vi "FTW-Endpoint-TCP-Receive-Worker.vi"(0 "TCP Endpoint":refnum<class "FTW-Endpoint-TCP.lvclass">, 5 "Address":string) -> ()   [LabVIEW 2013, in "FTW-Endpoint-TCP.lvclass"]
uses:
  FTW-Endpoint-TCP.lvclass
  FTW-Endpoint-TCP.lvclass/FTW-Endpoint-TCP.ctl
panel:
  out "connected":bool
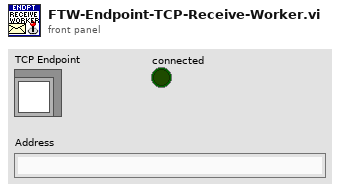
[diagram p1: front panel]
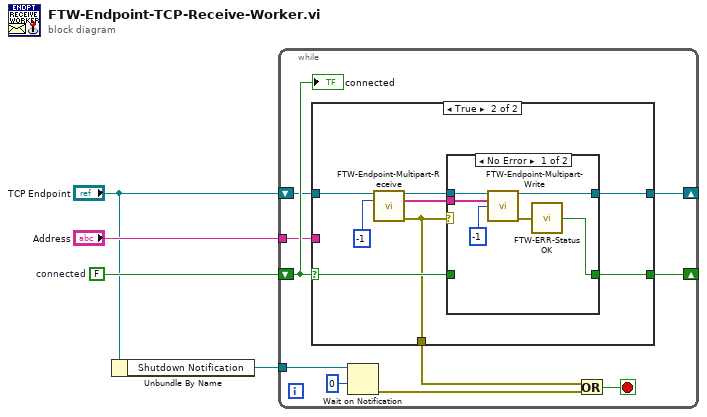
[diagram p0: block diagram]
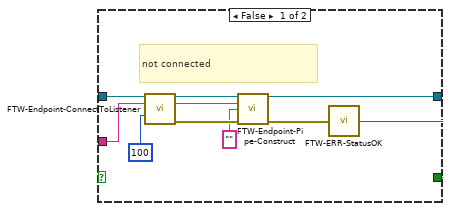
[diagram p2: hidden frame]
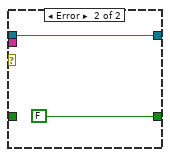
[diagram p3: hidden frame]
diagram:
  w4 = FALSE  # connected
  n1 = Unbundle By Name("TCP Endpoint") -> ("Shutdown Notification"=w1:refnum<notifier>)
  n2 = while {
    shift-right: [w11] -> _
    shift-left: w4 -> [w14]
    shift-right: [w12] -> _
    shift-left: "TCP Endpoint" -> [w7]
    tunnel: "Address" -> [w13]
    tunnel: w1 -> [w9]
    stop <- w6 stop-if-true
    n3 = case shown="True" w14 {
      selector: w14 -> [_ w29]
      tunnel: w13 -> [w24 _]
      tunnel: [w17 w31] -> w12
      tunnel: [w23 w30] -> w11
      tunnel: w7 -> [w20 w32]
      tunnel: [_ w27] -> w5
      frame False {
        # "not connected"
        n4 = call-dynamic "FTW-Endpoint-ConnectToListener.vi"("FTW-Endpoint In"=w20, "Address"=w24, "Timeout"=100) -> ("FTW-Endpoint Out"=w18:refnum<class "FTW-Endpoint-TCP.lvclass">, "Actual Address"=w16:string, "error out"=w22:errorcluster)  [unwired: 10 in]
        n5 = call-dynamic "FTW-Endpoint-Pipe-Construct.vi"("FTW Endpoint"=w18, "Address"=w16, "Requested Identity"="", "error in"=w22) -> ("FTW Endpoint out"=w17:refnum<class "FTW-Endpoint-TCP.lvclass">, "error out"=w19:errorcluster)  [unwired: 9 in, 1 out]
        n6 = call "FTW-ERR-StatusOK.vi"("error to check"=w19) -> ("Status OK?"=w23:bool)
      }
      frame True {
        n7 = call-dynamic "FTW-Endpoint-Multipart-Receive.vi"("FTW Endpoint"=w32, "Timeout"=-1) -> ("FTW Endpoint out"=w28:refnum<class "FTW-Endpoint-TCP.lvclass">, "Message Received"=w25:string[], "error out"=w27:errorcluster)  [unwired: 10 in, 1 out]
        n8 = case shown="No Error" w27 {
          tunnel: [w38 w40] -> w31
          tunnel: [w37 FALSE ("Status OK?")] -> w30
          tunnel: w29 -> [_ _]
          tunnel: w28 -> [w36 w40]
          tunnel: w25 -> [w35 _]
          frame No Error {
            n9 = call-dynamic "FTW-Endpoint-Multipart-Write.vi"("FTW Endpoint"=w36, "Multipart Message"=w35, "Timeout"=-1) -> ("FTW Endpoint out"=w38:refnum<class "FTW-Endpoint-TCP.lvclass">, "error out"=w34:errorcluster)  [unwired: 10 in, 1 out]
            n10 = call "FTW-ERR-StatusOK.vi"("error to check"=w34) -> ("Status OK?"=w37:bool)
          }
          frame Error {
          }
        }
      }
    }
    n11 = Wait on Notification(notifier=w9, timeout in ms (-1)=0) -> (error out=w8:errorcluster)  [unwired: 2 in, 3 out]
    n12 = Or(x=w5, y=w8) -> (x .or. y?=w6:bool)
    "connected" <- w14
  }
